vi "Build Tree Data.vi"(8 "error in (no error)":errorcluster, 11 "ITree Data in":refnum<class "ITree Data.lvclass">) -> (0 "error out":errorcluster, 3 "ITree Data out":refnum<class "ITree Data.lvclass">)   [LabVIEW 2020, in "Linked Lists.lvlib" / "ITree Data.lvclass"]
uses:
  <vilib>/gpm_packages/@cs/linked-list/Source/Tree Data/ITree Data/ITree Data.lvclass
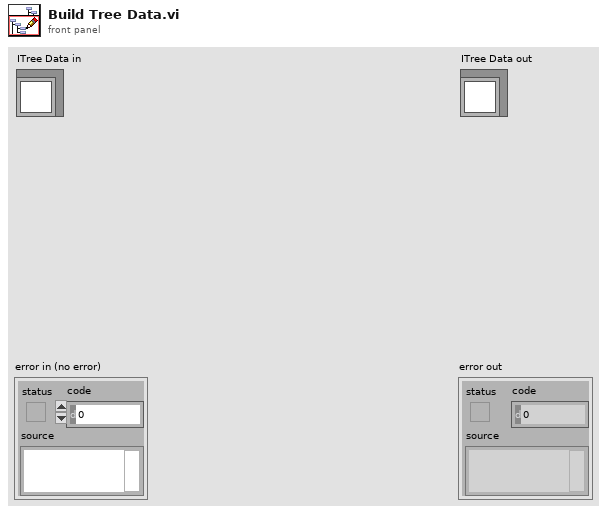
[diagram p1: front panel]
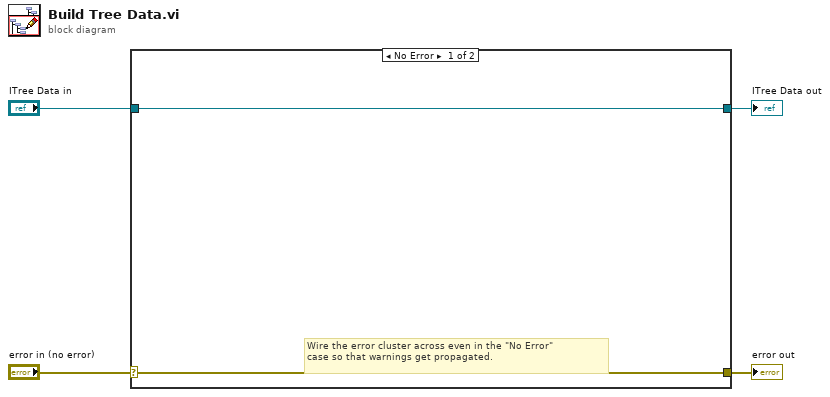
[diagram p0: block diagram]
diagram:
  n1 = case shown="No Error" "error in (no error)" {
    selector: "error in (no error)" -> [w5 w8]
    tunnel: [w5 w8] -> w3
    tunnel: [w6 w7] -> w1
    tunnel: "ITree Data in" -> [w6 w7]
    frame No Error {
      # "Wire the error cluster across even in the \"No Error\"\ncase so that warnings get propagated."
    }
    frame Error {
    }
  }
  "error out" <- w3
  "ITree Data out" <- w1
